vi "SQL查询.vi"(7 "condition":string, 10 "table输入":string(combo), 11 "database":string(combo)) -> (0 "error out":errorcluster, 3 "data":string[][](table))   [LabVIEW 2016]
uses:
  <vilib>/Utility/sysdir.llb/System Directory Type.ctl
  <vilib>/addons/database/Connection.llb/DB Tools Open Connec (String).vi
  <vilib>/addons/database/_DB Variant To Data/Database Variant To Data.xnode
  <vilib>/addons/database/NI_Database_API.lvlib
panel:
  in  "error in (no error)":errorcluster
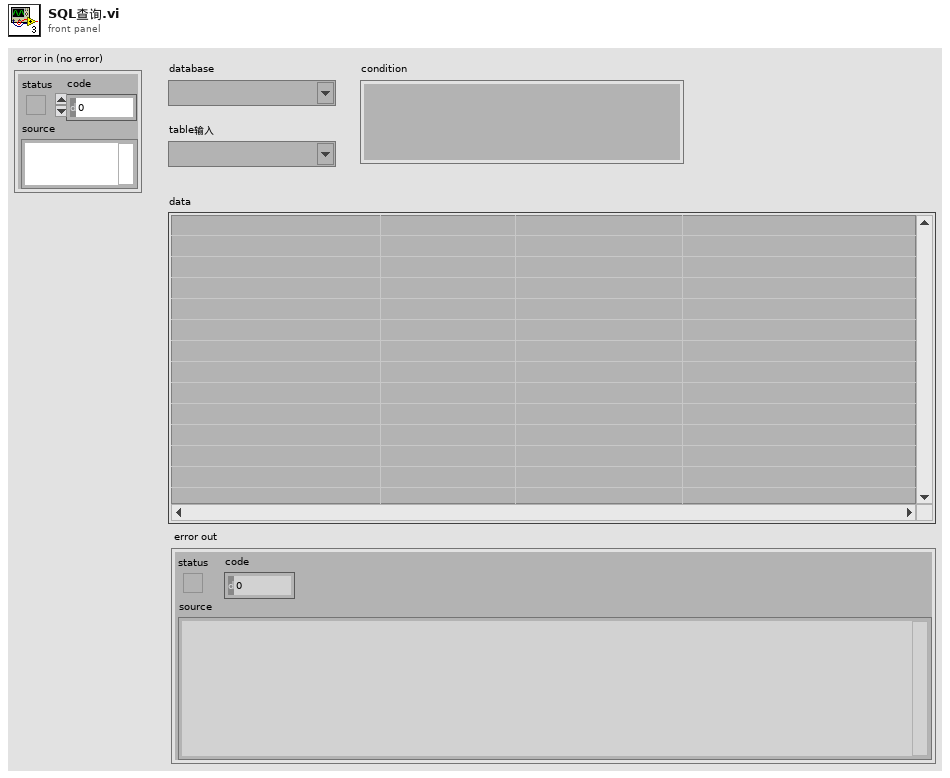
[diagram p1: front panel]
types:
  T1 = typedef "System Directory Type.ctl" = i32
  T2 = typedef "NI_Database_API.lvlib/Conn ObjectReference.ctl" = refnum<k1>
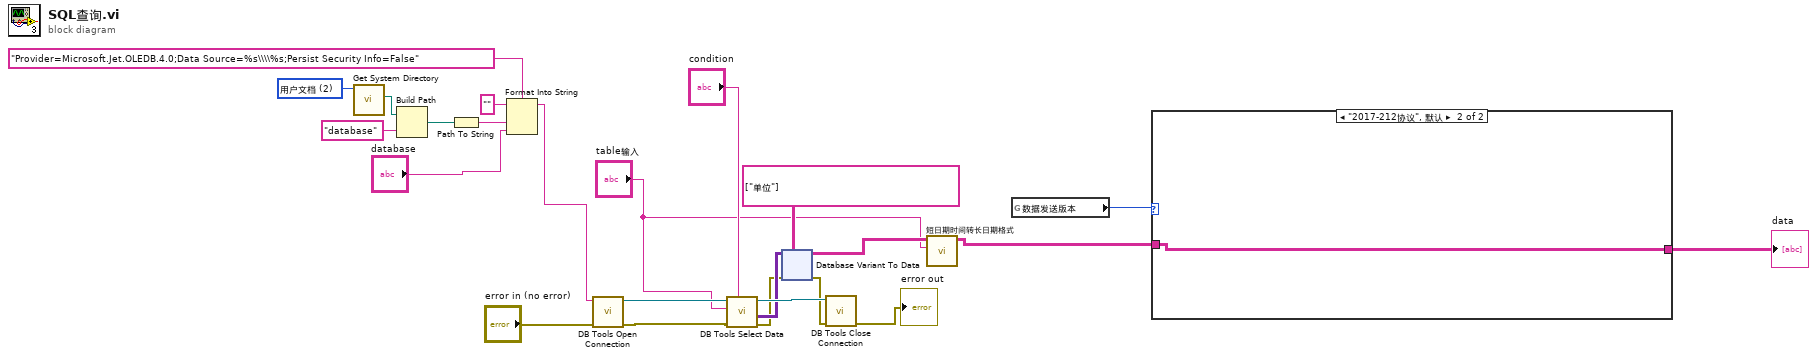
[diagram p0: block diagram]
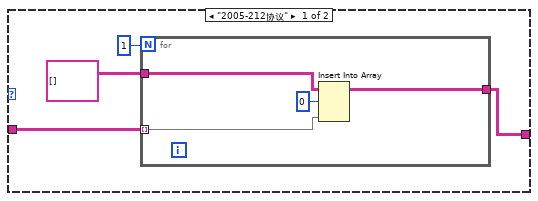
[diagram p2: hidden frame]
diagram:
  w17 = T1 2 items=["用户目录"=0, "用户桌面"=1, "用户文档"=2, "用户应用程序数据"=3, "用户设置"=4, "用户临时目录"=5, "公共文档"=6, "公共应用程序数据"=7, "公共设置"=8, "公共缓存"=13, "系统核心库"=9, "系统安装库"=10, "应用程序文件"=11, "启动盘根目录"=12] ("system directory type")
  n1 = call <vilib>:"Get System Directory.vi"("system directory type"=w17) -> ("system directory"=w18:path)  [unwired: 10 in]
  n2 = Build Path(base path=w18, name or relative path="database" ("condition")) -> (appended path=w20:path)
  n3 = Path To String(path=w20) -> (string=w16:string)
  n4 = Format Into String(format string="Provider=Microsoft.Jet.OLEDB.4.0;Data Source=%s\\\\%s;Persist Security Info=False" ("格式字符串"), initial string="" ("初始字符串"), w16, "database") -> (resulting string=w8:string)  [unwired: 1 in, 1 out]
  n5 = call-poly <vilib>:"DB Tools Open Connection.vi"("error in (no error)"="error in (no error)", "connection information"=w8) -> ("error out"=w6:errorcluster, "connection reference"=w7:T2)  [unwired: 6 in]
  n6 = call <vilib>:"DB Tools Select Data.vi"("condition"="condition", "error in (no error)"=w6, "table"="table输入", "connection reference"=w7) -> ("error out"=w13:errorcluster, "data"=w23:variant[][], "connection reference out"=w24:T2)  [unwired: 2 in]
  n7 = xnode "Database Variant To Data"("database variant"=w23, "error in (no error)"=w13, "type"=string[][] [["单位"]]) -> ("data"=w5:string[][], "error out"=w12:errorcluster)
  n8 = call <vilib>:"DB Tools Close Connection.vi"("error in (no error)"=w12, "connection reference"=w24) -> ("error out"=→"error out":errorcluster)  [unwired: 5 in]
  n9 = call "短日期时间转长日期格式.vi"("table输入"="table输入", "data"=w5) -> ("输出数组"=w2:string[][])  [unwired: 9 in]
  n10 = global read "全局1.vi" "数据发送版本"() -> (w3:enum16{"2005-212协议", "2017-212协议"})
  n11 = case shown="\"2017-212协议\", 默认" w3 {
    tunnel: w2 -> [w26 w33]
    tunnel: [w25 w33] -> w1
    frame "2005-212协议" {
      n12 = for {
        N: 1 -> [_]
        tunnel: string[][] [] ("data") -> [w32]
        tunnel: w26 -> [w31] mode=indexing
        tunnel: [w29] -> w25
        n13 = Insert Into Array(array=w32, index (row)=0 ("索引 (行)"), new element=w31) -> (w29:string[][])  [unwired: 1 in]
      }
    }
    frame "2017-212协议", Default {
    }
  }
  "data" <- w1
